vi "ET2604 - Read Humidity.vi"(8 "error in (no error)":errorcluster, 11 "VISA resource name":refnum<visa-resource-name>) -> (0 "error out":errorcluster, 2 "Data":sgl, 3 "VISA resource name out":refnum<visa-resource-name>)   [LabVIEW 2017]
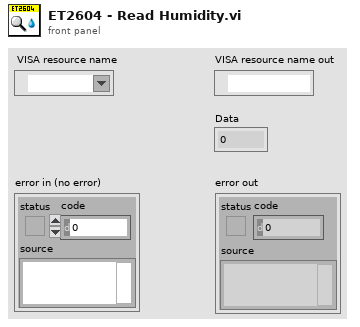
[diagram p1: front panel]
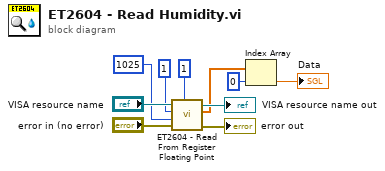
[diagram p0: block diagram]
diagram:
  n1 = call "ET2604 - Read From Register Floating Point.vi"("Num Of Reg (1)"=u16 1, "error in (no error)"="error in (no error)", "Register Address (0)"=u16 1025, "Unit Address (1)"=u8 1, "VISA session"="VISA resource name") -> ("error out"=→"error out":errorcluster, "Data"=w3:sgl[], "dup VISA session"=→"VISA resource name out":refnum<visa-resource-name>)  [unwired: 4 in]
  n2 = Index Array(array=w3, index=0) -> (element=→"Data":sgl)
